vi "Ping.vi"(6 "timeout (ms)":i32=5000, 8 "error in":errorcluster, 11 "gRPC ID in":T3) -> (0 "error out":errorcluster, 2 "loader_info":T1, 3 "gRPC ID out":T3)   [LabVIEW 2021, in "CIFPluginLoaderClientWrapper.lvlib"]
uses:
  CIFPluginLoaderClientWrapper.lvlib
  <vilib>/gRPC/LabVIEW gRPC Library/Shared/grpcId.ctl
  CIF_PluginLoader_client/RPC Messages/cif_management_common_LoaderInfoFull.ctl
  CIF_PluginLoader_client/RPC Messages/cif_management_common_LoaderType.ctl
  CIF_PluginLoader_client/RPC Messages/cif_pluginloader_PingRequest.ctl
  CIF_PluginLoader_client/CIF_PluginLoader_client.lvlib
  <vilib>/gRPC/LabVIEW gRPC Library/grpc-lvsupport-release.lvlib
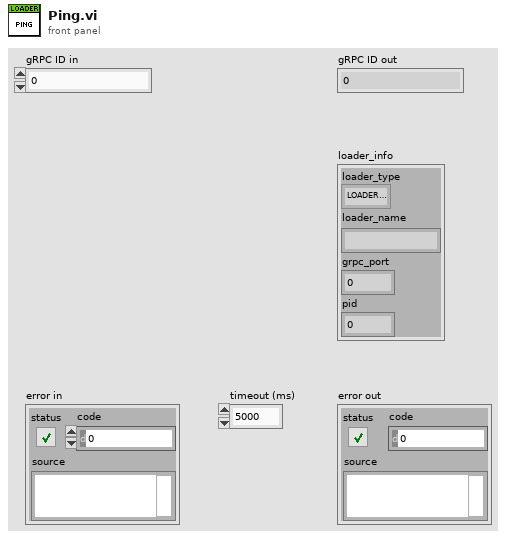
[diagram p1: front panel]
types:
  T1 = typedef "CIF_PluginLoader_client.lvlib/cif_management_common_LoaderInfoFull.ctl" = cluster{"loader_type":T2, "loader_name":string, "grpc_port":i32, "pid":u32}
  T2 = typedef "CIF_PluginLoader_client.lvlib/cif_management_common_LoaderType.ctl" = enum32{"LOADERTYPE_UNKNOWN", "LOADERTYPE_LABVIEW"}
  T3 = typedef "grpc-lvsupport-release.lvlib/grpcId.ctl" = u64
  T4 = typedef "CIF_PluginLoader_client.lvlib/cif_pluginloader_PingRequest.ctl" = cluster{"void":string}
  T5 = typedef "CIF_PluginLoader_client.lvlib/cif_pluginloader_PingResponse.ctl" = cluster{"loader_info":T1}
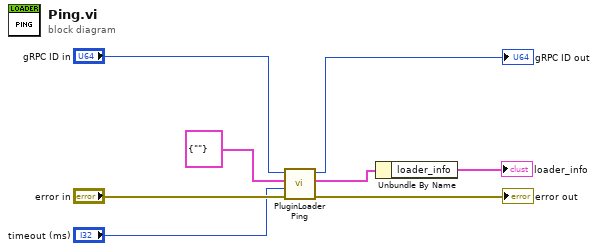
[diagram p0: block diagram]
diagram:
  n1 = call "PluginLoader Ping.vi"("error in"="error in", "timeout (ms)"="timeout (ms)", "Request Data"=T4 {"void"=""}, "gRPC ID"="gRPC ID in") -> ("error out"=→"error out":errorcluster, "Response Data"=w2:T5, "gRPC ID out"=→"gRPC ID out":T3)  [unwired: 5 in]
  n2 = Unbundle By Name(w2) -> ("loader_info"=→"loader_info":T1)
